vi "Untitled 1.vi"() -> ()   [LabVIEW 2013]
uses:
  <vilib>/measure/mamon.llb/Waveform Peak Detection for N Chan.vi
  DAQ_global.vi
  <vilib>/measure/madcrms.llb/Basic Averaged DC-RMS for N Chan.vi
  <vilib>/express/express analysis/Spectral/Block/exnSpectralBlock spectral measurements peak poly.vi
  <vilib>/express/express analysis/Spectral/Block/exnSpectralBlock spectral measurements peak DDT.vi
  <vilib>/express/express analysis/Spectral/XNode/ExpressSpectralMeasurementsBlockNode.xnode
  <vilib>/measure/NI_MAPro.lvlib
panel:
  out "Amplitudes":cluster{"Amplitudes":dbl[]}[](array[cluster]) {"Amplitudes" format="%.2p"}
  out "RMS values":dbl[](array[numeric]) format="%.2p"
  in  "rate":dbl=100000.0
  in  "number of samples":i32=10000
  out "THD":dbl
  out "Frequency":dbl
  out "Amplitude":dbl
  out "Spectrum":dynamicdata(graph)
  out "data":dynamicdata(graph) caption="Waveform"
  in  "stop":bool
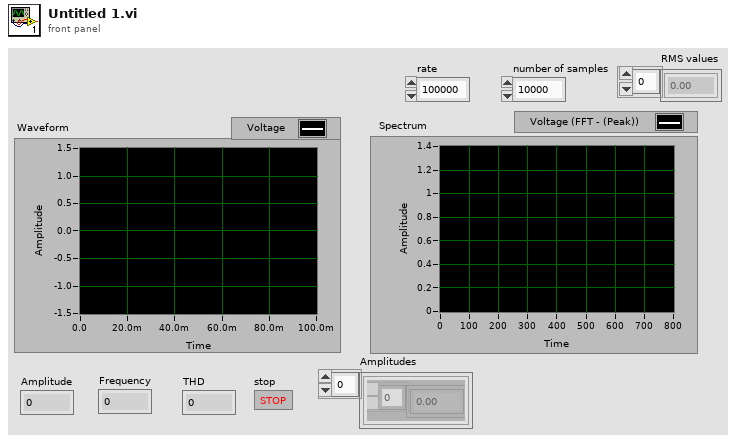
[diagram p1: front panel]
types:
  T1 = cluster{"averaging mode":u16, "weighting mode":u16, "number of averages":u32}
  T2 = cluster{"dB On (F)":bool, "unwrap phase (F)":bool, "convert to degree (F)":bool}
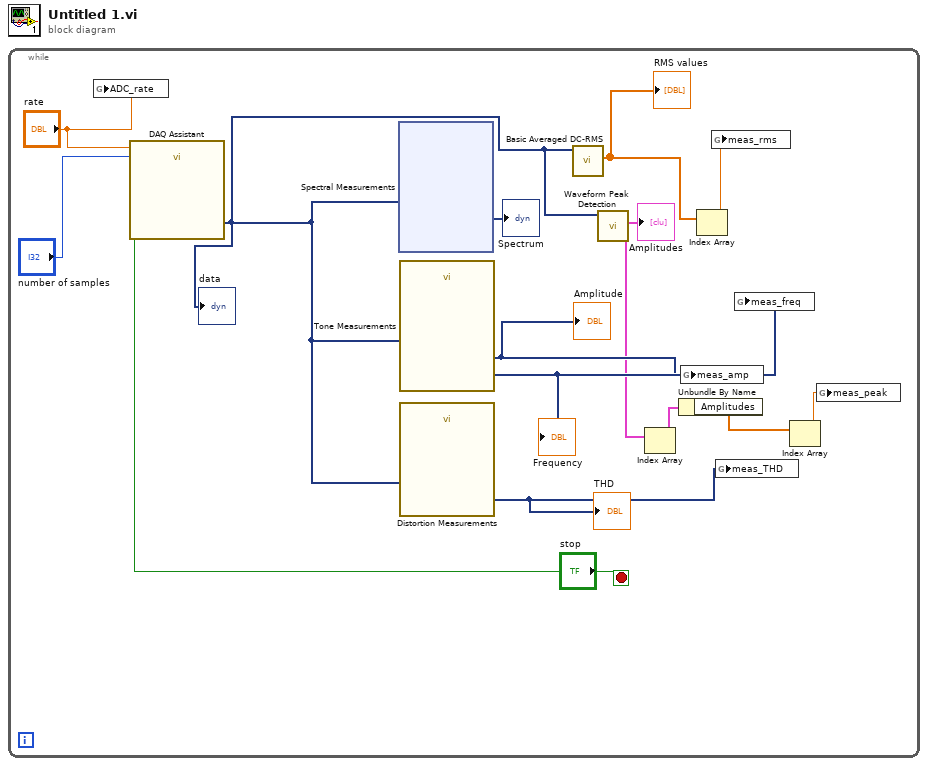
[diagram p0: block diagram]
diagram:
  n1 = while {
    stop <- "stop" stop-if-true
    n2 = global write "DAQ_global.vi" "ADC_rate"("rate") -> ()
    n3 = call "DAQ Assistant"("rate"="rate", "number of samples"="number of samples", "stop (T)"="stop") -> ("data"=w11:dynamicdata)  [unwired: 14 in, 2 out]
    "data" <- w11
    n4 = xnode "Spectral Measurements"("Signals"=w11) -> ("FFT - (Peak)"=→"Spectrum":dynamicdata)  [unwired: 1 in, 2 out]
    n5 = call "Tone Measurements"("Signals"=w11) -> ("Frequency"=w8:dynamicdata, "Amplitude"=w7:dynamicdata)  [unwired: 8 in, 1 out]
    "Amplitude" <- w7
    "Frequency" <- w8
    n6 = call "Distortion Measurements"("Signals"=w11) -> ("THD"=w9:dynamicdata)  [unwired: 9 in, 1 out]
    "THD" <- w9
    n7 = call-poly <vilib>:"Basic Averaged DC-RMS.vi"("signals in"=w11) -> ("RMS values"=w2:dbl[])  [unwired: 7 in, 3 out]
    "RMS values" <- w2
    n8 = call-poly <vilib>:"Waveform Peak Detection.vi"("Signals In"=w11) -> ("Amplitudes"=w6:cluster{"Amplitudes":dbl[]}[])  [unwired: 6 in, 4 out]
    "Amplitudes" <- w6
    n9 = Index Array(array=w6) -> (element=w5:cluster{"Amplitudes":dbl[]})  [unwired: 1 in]
    n10 = Unbundle By Name(w5) -> ("Amplitudes"=w4:dbl[])
    n11 = global write "DAQ_global.vi" "meas_amp"(w7) -> ()
    n12 = Index Array(array=w2) -> (element=w1:dbl)  [unwired: 1 in]
    n13 = global write "DAQ_global.vi" "meas_rms"(w1) -> ()
    n14 = global write "DAQ_global.vi" "meas_THD"(w9) -> ()
    n15 = global write "DAQ_global.vi" "meas_freq"(w8) -> ()
    n16 = Index Array(array=w4) -> (element=w3:dbl)  [unwired: 1 in]
    n17 = global write "DAQ_global.vi" "meas_peak"(w3) -> ()
  }
